vi "Turnrate_to_Side_Drag.vi"(1 "Current Turn Rate":dbl[](array[numeric]) format="%_6g") -> (0 "Current Drag":dbl[](array[numeric]) format="%_6g")   [LabVIEW 2009]
uses:
  <vilib>/gmath/NI_Gmath.lvlib
panel:
  in  "Drag / Turn Rate":cluster{"F":dbl, "V":dbl}[](array[cluster])
  # "Drag is in N\nTurn Rate in deg/s"
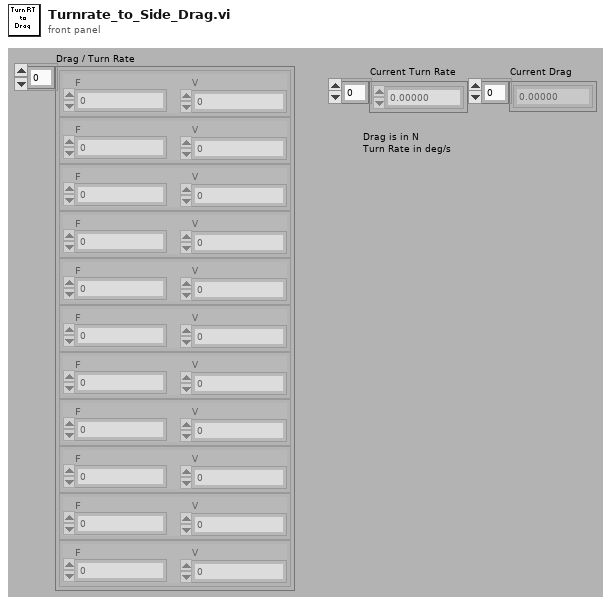
[diagram p1: front panel]
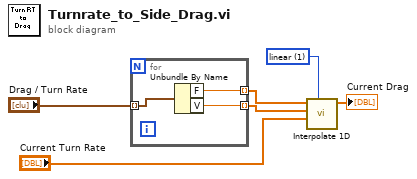
[diagram p0: block diagram]
diagram:
  w6 = 1 items=["nearest", "linear", "spline", "cubic Hermite", "Lagrange"] ("method")
  n1 = for {
    tunnel: "Drag / Turn Rate" -> [w9] mode=indexing
    tunnel: [w8] -> w4 mode=indexing
    tunnel: [w7] -> w3 mode=indexing
    n2 = Unbundle By Name(w9) -> ("F"=w8:dbl, "V"=w7:dbl)
  }
  n3 = call <vilib>:"Interpolate 1D.vi"("method"=w6, "xi"="Current Turn Rate", "X"=w3, "Y"=w4) -> ("yi"=→"Current Drag":dbl[])  [unwired: 5 in, 2 out]
